vi "Limits(DoubleEncoder).vi"(4 "Into Home Limit is Pos (Encoder)":bool=TRUE, 5 "Encoder Limit":dbl format="%#_13g", 6 "Into Home Limit Is Pos (Motor)":bool, 7 "Home Encoder Limit":dbl format="%#_13g", 8 "Power In":dbl format="%#_13g", 10 "Motor Ref":T1={"DeviceStatus"={"status"=FALSE, "code"=0, "source"=""}, "Type"=enum."PWM", "PWM"={"PWM Channel"=enum."Invalid", "DeadBand"={"Name"="", "maxPositivePwm"=0, "minPositivePwm"=0, "centerPwm"=0, "maxNegativePwm"=0, "minNegativePwm"=0, "angularRange"=0}}, "CAN"={"Device Number"=0, "SetOutput VI Ref"=variant, "GetOutput VI Ref"=variant, "Enable VI Ref"=variant, "Disable VI Ref"=variant, "Data"=variant}, "Invert"=FALSE, "DIO PWM"={"PWM \"Enable\" Channel"=enum."Invalid", "DIOChannel"=enum."Invalid", "PWM Rate"=0.0}}) -> (0 "Power Out":dbl)   [LabVIEW 2018]
uses:
  <vilib>/Rock Robotics/WPI/MotorControl/WPI_MotorControlDeviceRef.ctl
  <vilib>/Rock Robotics/WPI/MotorControl/WPI_MotorControlType.ctl
  <vilib>/Rock Robotics/SystemInterfaces/DIO/FPGA_DIOPWMChannel.ctl
  <vilib>/Rock Robotics/WPI/PWM/WPI_PWMDeadband.ctl
  <vilib>/Rock Robotics/SystemInterfaces/DIO/FPGA_DIOChannel.ctl
  <vilib>/Rock Robotics/WPI/ThirdParty/Phoenix-LabVIEW/Motor Controller/Get/CTRE_Phoenix_MotorController_GetSelectedSensorData.vi
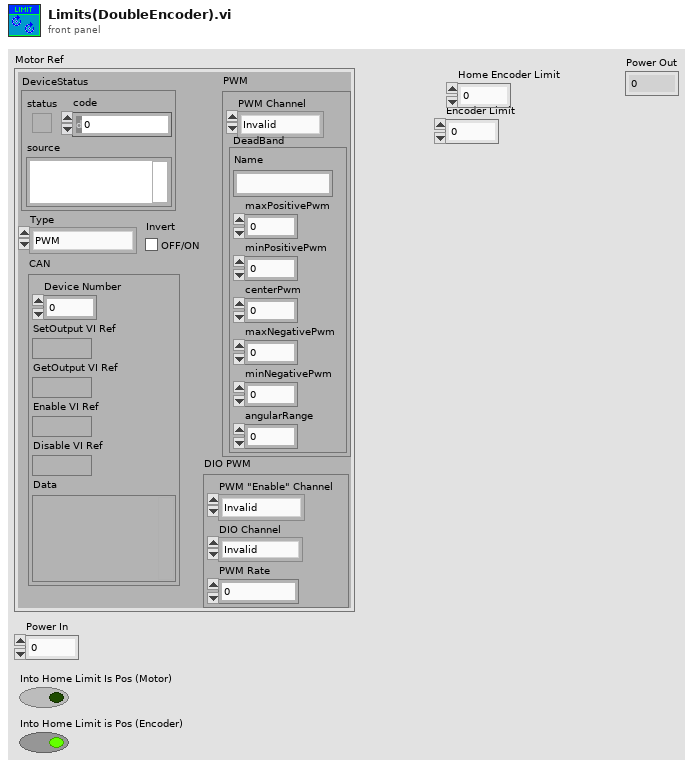
[diagram p1: front panel]
types:
  T1 = typedef "WPI_MotorControlDeviceRef.ctl" = cluster{"DeviceStatus":errorcluster, "Type":T2, "PWM":cluster{"PWM Channel":T3, "DeadBand":T4}, "CAN":cluster{"Device Number":u8, "SetOutput VI Ref":variant, "GetOutput VI Ref":variant, "Enable VI Ref":variant, "Disable VI Ref":variant, "Data":variant}, "Invert":bool, "DIO PWM":cluster{"PWM \"Enable\" Channel":T3, "DIOChannel":T5, "PWM Rate":dbl}}
  T2 = typedef "WPI_MotorControlType.ctl" = enum16{"PWM", "CAN", "DIO PWM"}
  T3 = typedef "FPGA_DIOPWMChannel.ctl" = enum8{"PWM 0", "PWM 1", "PWM 2", "PWM 3", "PWM 4", "PWM 5", "PWM 6", "PWM 7", "PWM 8", "PWM 9", "PWM MXP 0", "PWM MXP 1", "PWM MXP 2", "PWM MXP 3", "PWM MXP 4", "PWM MXP 5", "PWM MXP 6", "PWM MXP 7", "PWM MXP 8", "PWM MXP 9", "Invalid"}
  T4 = typedef "WPI_PWMDeadband.ctl" = cluster{"Name":string, "maxPositivePwm":i32, "minPositivePwm":i32, "centerPwm":i32, "maxNegativePwm":i32, "minNegativePwm":i32, "angularRange":u16}
  T5 = typedef "FPGA_DIOChannel.ctl" = enum8{"DIO 0", "DIO 1", "DIO 2", "DIO 3", "DIO 4", "DIO 5", "DIO 6", "DIO 7", "DIO 8", "DIO 9", "DIO MXP 0", "DIO MXP 1", "DIO MXP 2", "DIO MXP 3", "DIO MXP 4", "DIO MXP 5", "DIO MXP 6", "DIO MXP 7", "DIO MXP 8", "DIO MXP 9", "DIO MXP 10", "DIO MXP 11", "DIO MXP 12", "DIO MXP 13", "DIO MXP 14", "DIO MXP 15", "SPI Port CS1", "SPI Port CS2", "SPI Port CS3", "SPI Port MISO", "SPI Port MOSI", "Invalid"}
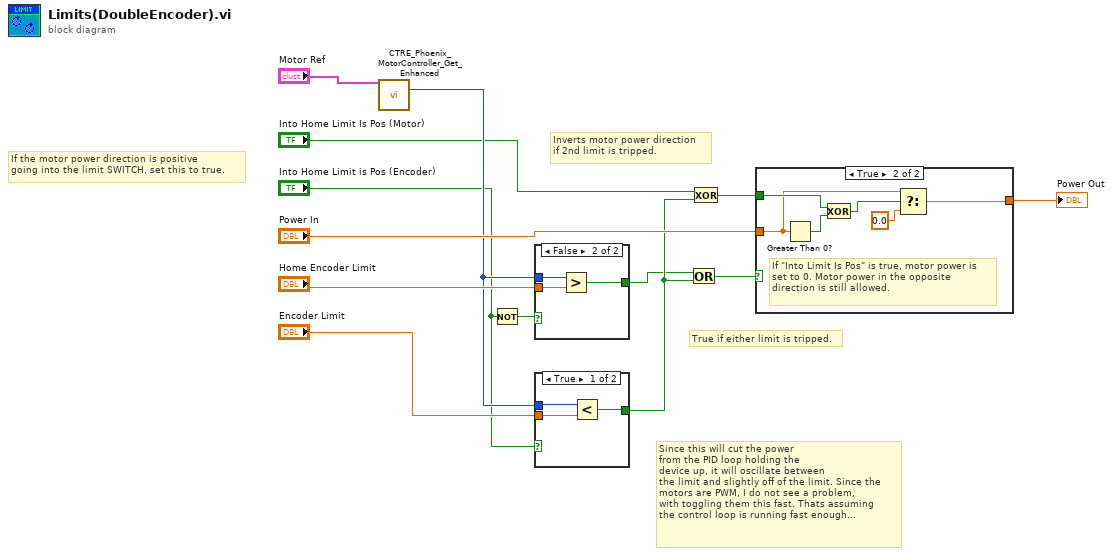
[diagram p0: block diagram]
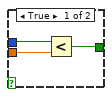
[diagram p2: hidden frame]
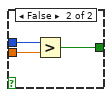
[diagram p3: hidden frame]
diagram:
  # "True if either limit is tripped."
  # "Inverts motor power direction\nif 2nd limit is tripped."
  # "Since this will cut the power\nfrom the PID loop holding the\ndevice up, it will oscillate between\nthe limit and slightly off of the limit. Since the\nmotors are PWM, I do not see a problem,\nwith toggling them this fast. Thats assuming\nthe control loop is running fast enough..."
  # "If the motor power direction is positive\ngoing into the limit SWITCH, set this to true."
  n1 = call-poly <vilib>:"CTRE_Phoenix_MotorController_Get_Enhanced.vi"("PhoenixMotorControlDevRef"="Motor Ref") -> ("Position (Raw Sensor Units)"=w5:i32)  [unwired: 11 in, 3 out]
  n2 = Not(x="Into Home Limit is Pos (Encoder)") -> (.not. x?=w4:bool)
  n3 = case shown="False" w4 {
    tunnel: "Home Encoder Limit" -> [w14 w19]
    tunnel: w5 -> [w15 w18]
    tunnel: [w16 w17] -> w3
    frame True {
      n4 = Less?(x=w15, y=w14) -> (x < y?=w16:bool)
    }
    frame False {
      n5 = Greater?(x=w18, y=w19) -> (0:w17:bool)
    }
  }
  n6 = case shown="True" "Into Home Limit is Pos (Encoder)" {
    tunnel: "Encoder Limit" -> [w20 w25]
    tunnel: w5 -> [w21 w24]
    tunnel: [w22 w23] -> w7
    frame True {
      n7 = Less?(x=w21, y=w20) -> (x < y?=w22:bool)
    }
    frame False {
      n8 = Greater?(x=w24, y=w25) -> (0:w23:bool)
    }
  }
  n9 = Or(x=w3, y=w7) -> (x .or. y?=w10:bool)
  n10 = Exclusive Or(1:w7, 2:"Into Home Limit Is Pos (Motor)") -> (0:w9:bool)
  n11 = case shown="True" w10 {
    tunnel: [w26 w29] -> w12
    tunnel: w9 -> [_ w28]
    tunnel: "Power In" -> [w26 w27]
    frame False {
    }
    frame True {
      # "If \"Into Limit Is Pos\" is true, motor power is set to 0. Motor power in the opposite direction is still allowed."
      n12 = Greater Than 0?(x=w27) -> (x > 0?=w31:bool)
      n13 = Exclusive Or(1:w31, 2:w28) -> (0:w30:bool)
      n14 = Select(t=w27, s=w30, f=0.0) -> (s? t:f=w29:dbl)
    }
  }
  "Power Out" <- w12
